vi "Host_Test_output_DDS.vi"() -> ()   [LabVIEW 2013]
uses:
  <vilib>/rvi/interface/nirviOpenFPGA/nirviOpenFPGA.xnode
  FPGA Bitfiles/FPGAoutputfromDDS_d89QWMi772M.lvbitx
  FPGAoutput_from_DDS.vi
  <vilib>/FPGAPlugInAG/PXIe-7975R/niLvFpga_Open_PXIe-7975R.vi
  <vilib>/rvi/interface/common/dynamic/niFpgaDynamicAddResources.vi
  <vilib>/rvi/interface/nirviReadWriteControl/nirviReadWriteControl.xnode
  NiFpgaLv.dll
  <vilib>/Utility/error.llb/Error Cluster From Error Code.vi
  <vilib>/rvi/interface/Simulation/niFpgaSimulationCallBeginRW.vi
  <vilib>/rvi/errors/niLvFpgaAdjustHostInterfaceError.vi
  <vilib>/rvi/interface/nirviCloseFPGA/nirviCloseFPGA.xnode
  <vilib>/FPGAPlugInAG/Dynamic/niLvFpga_Close_Dynamic.vi
  <vilib>/userdefined/High Color/nirio_resource_hc.ctl
panel:
  in  "Output mixer fequency [MHz]":dbl
  in  "stop":bool
  out "Configured?":bool
  out "Clocking Option Configured?":bool
  in  "resource name":T1="RIO0"
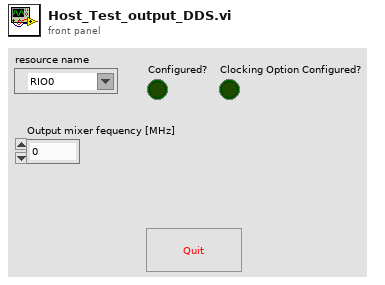
[diagram p1: front panel]
types:
  T1 = typedef "nirio_resource_hc.ctl" = tag
  T2 = enum8{"Internal Clock PLL Off", "Internal Clock PLL On (REF IN)", "External Clock (CLK_IN)", "Internal Clock PLL On (IoModSyncClk)"}
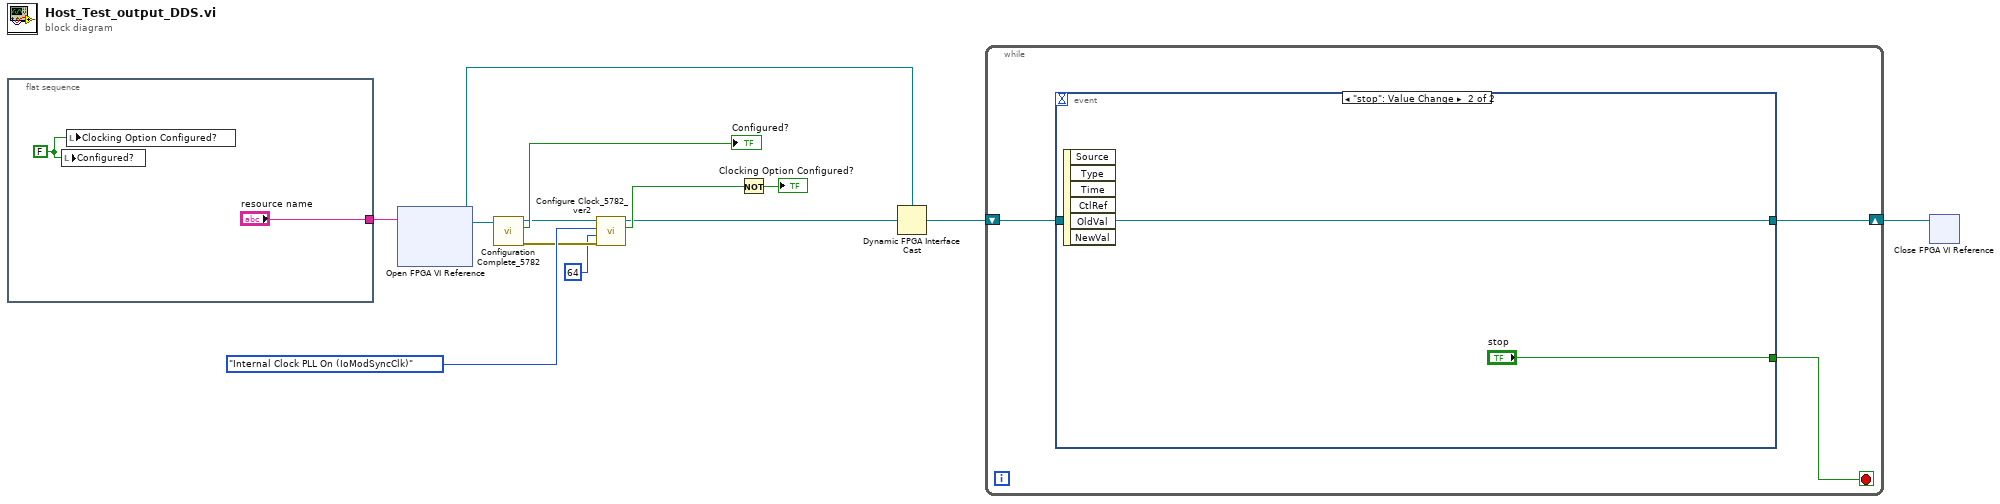
[diagram p0: block diagram]
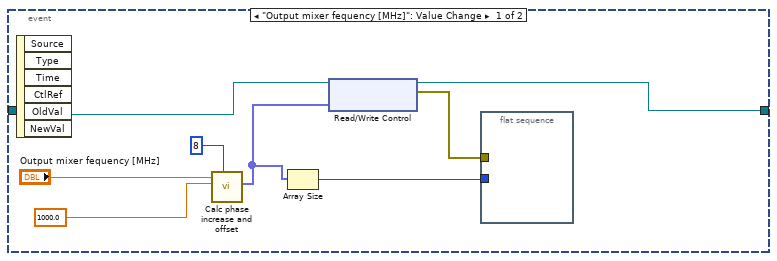
[diagram p2: hidden frame]
diagram:
  n1 = flat-sequence {
    tunnel: ["resource name"] -> w12
    frame #0 {
      w13 = FALSE ("Trigger Acquisition")
      n2 = local write "Configured?"(w13) -> ()
      n3 = local write "Clocking Option Configured?"(w13) -> ()
    }
  }
  n4 = xnode "Open FPGA VI Reference"("resource name"=w12) -> ("FPGA VI Reference Out"=w3:refnum<k20>)  [unwired: 1 in, 1 out]
  n5 = call "Configuration Complete_5782.vi"("FPGA VI Reference in"=w3) -> ("error out"=w7:errorcluster, "Configured?"=→"Configured?":bool, "FPGA VI Reference out"=w6:refnum<k20>)  [unwired: 8 in]
  n6 = call "Configure Clock_5782_ver2.vi"("error in"=w7, "User Data 1"=u8 64, "Clock Source"=T2."Internal Clock PLL On (IoModSyncClk)", "FPGA VI Reference"=w6) -> ("Configuration Error"=w10:bool, "FPGA VI Reference out"=w4:refnum<k20>)  [unwired: 5 in, 1 out]
  n7 = Not(x=w10) -> (.not. x?=→"Clocking Option Configured?":bool)
  n8 = Dynamic FPGA Interface Cast(Session In=w3, Type=w4) -> (Session Out=w2:refnum<k20>)
  n9 = while {
    shift-right: [w16] -> w1
    shift-left: w2 -> [w17]
    stop <- w15 stop-if-true
    n10 = event shown="[1] \"stop\": Value Change" {
      selector: _ -> [_ _]
      dyn-events: _ -> [_ _]
      timeout: _ -> [_ _]
      tunnel: w17 -> [w20 w27]
      tunnel: [w19 w27] -> w16
      tunnel: [_ "stop"] -> w15
      event "Output mixer fequency [MHz]": Value Change {
        n11 = event-data() -> ()  [unwired: 1 in, 6 out]
        n12 = call "Calc phase increase and offset.vi"("# of DDS"=8, "fclk (MHz)"=1000.0 ("fclk (800MHz)"), "f_generated (MHz)"="Output mixer fequency [MHz]") -> ("Phase out"=w22:fxp<+,64,64>[])  [unwired: 6 in, 2 out]
        n13 = Array Size(array=w22) -> (size(s)=w23:i32)
        n14 = xnode "Read/Write Control"("FPGA VI Reference In"=w20, "Phase output"=w22) -> ("FPGA VI Reference Out"=w19:refnum<k20>, "error out"=w21:errorcluster)  [unwired: 1 in]
        n15 = flat-sequence {
          tunnel: w21 -> [_]
          tunnel: w23 -> [_]
          frame #0 {
          }
        }
      }
      event "stop": Value Change {
        n16 = event-data() -> ()  [unwired: 1 in, 6 out]
      }
    }
  }
  n17 = xnode "Close FPGA VI Reference"("FPGA VI Reference In"=w1) -> ()  [unwired: 1 in, 1 out]
